vi "raise move v0.5.vi"(8 "error in (no error)":errorcluster) -> (0 "error out":errorcluster)   [LabVIEW 2019]
uses:
  <vilib>/Platform/TimedLoop/XDataNode/timing_clust.ctl
  <vilib>/Platform/TimedLoop/XDataNode/nitl_modes.ctl
  <vilib>/Platform/TimedLoop/XDataNode/wakeup.ctl
  FPGA_subVIs/low level/motor/motor enum.ctl
  <vilib>/platform/TimedLoop/XDataNode/XDataNode.xnode
  <vilib>/Platform/TimedLoop/XDataNode/XDNodeRunTimeDep.lvlib
  FPGA_subVIs/low level/motor/motor.lvlib
panel:
  out "Numeric":dbl
  out "-x":dbl
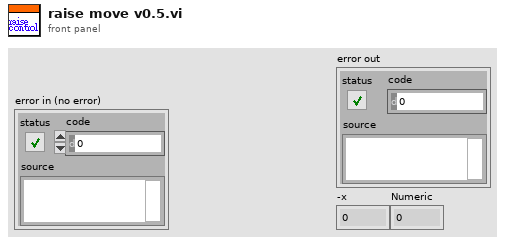
[diagram p1: front panel]
types:
  T1 = typedef "XDNodeRunTimeDep.lvlib/timing_clust.ctl" = cluster{"Expected End [f-1]":u64, "Actual End [f-1]":u64, "Finished Late? [f-1]":bool, "Expected End [i-1]":u64, "Actual End [i-1]":u64, "Finished Late? [i-1]":bool, "Expected Start [i]":u64, "Actual Start [i]":u64, "Expected Start [f]":u64, "Actual Start [f]":u64, "Source Name":string, "Structure Name":string, "Period":i64, "Deadline":i64, "Offset":i64, "Start":i64, "Priority":i32, "Timeout":i32, "Mode":T2, "Wakeup Reason":T3, "Error":errorcluster, "Source Type":string, "Secondary Source Type":string, "Global End Time":u64, "Global Start Time":u64, "Frame Duration":u64, "Iteration Duration":u64, "Assigned CPU":i32, "I/O Scan Engine Mode":u32}
  T2 = typedef "XDNodeRunTimeDep.lvlib/nitl_modes.ctl" = enum32{"No Change", "Process missed periods, maintain original phase", "Discard missed periods, maintain original phase", "Process missed periods, ignore original phase", "Discard missed periods, ignore original phase"}
  T3 = typedef "XDNodeRunTimeDep.lvlib/wakeup.ctl" = enum32{"Normal", "Aborted", "Asynchronous wakeup", "Timing source error", "Timed loop error", "Timeout"}
  T4 = typedef "my FPGA lib.lvlib/motor.lvlib/motor enum.ctl" = enum16{"M1", "M2", "M3", "M4"}
  T5 = cluster{"proportional gain (Kc)":dbl, "integral time (Ti, min)":dbl, "derivative time (Td, min)":dbl}
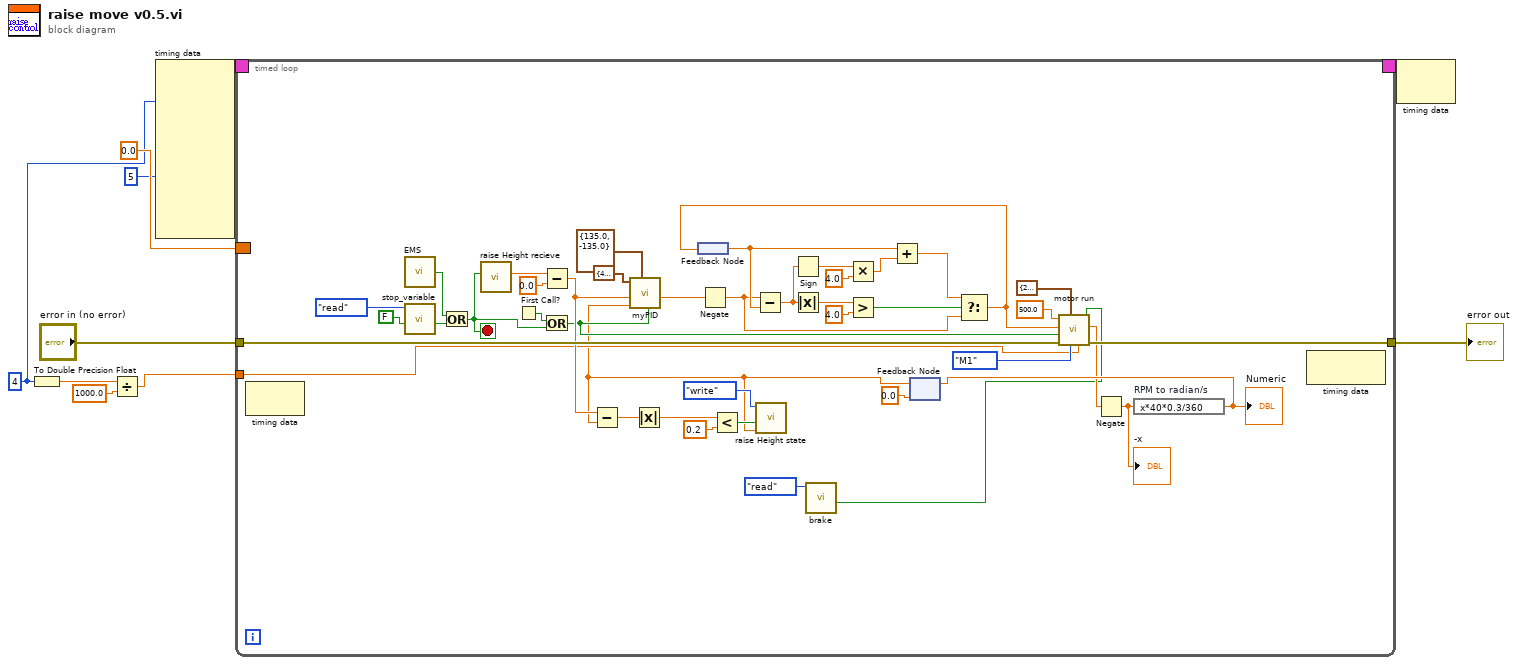
[diagram p0: block diagram]
diagram:
  w4 = i64 4 ("Period")
  n1 = To Double Precision Float(number=w4) -> (double precision float=w8:dbl)
  n2 = Divide(x=w8, y=1000.0) -> (x/y=w3:dbl)
  n3 = node-c288(w4, i64 5 ("Offset")) -> (w10:T1)  [unwired: 8 in]
  n4 = timed-loop {
    timing: w10 -> [_]
    timing-out: [_] -> w9
    tunnel: w3 -> [w18]
    tunnel: [w48] -> w6
    border: 0.0 -> [_]
    tunnel: "error in (no error)" -> [w34]
    stop <- w14 stop-if-true
    n5 = node-c288() -> ()  [unwired: 1 in, 1 out]
    n6 = call "EMS.vi"() -> ("A/DIO4 (Pin 19)"=w32:bool)
    n7 = call "stop_variable.vi"("Write"=FALSE, "Enum"=enum16{"read", "write"}."read") -> ("read"=w30:bool)  [unwired: 8 in, 1 out]
    n8 = Or(x=w32, y=w30) -> (x .or. y?=w14:bool)
    n9 = call "raise Height recieve.vi"("stop?"=w14) -> ("Height_cm"=w37:dbl)  [unwired: 9 in, 1 out]
    n10 = First Call?() -> (First Call?: T/F=w19:bool)
    n11 = Subtract(x=w37, y=0.0 ("x")) -> (x-y=w29:dbl)
    n12 = Or(x=w19, y=w14) -> (x .or. y?=w15:bool)
    n13 = feedback #1() -> (w44:dbl)
    n14 = call "brake.vi"("Enum"=enum16{"read", "write"}."read") -> ("read"=w12:bool)  [unwired: 9 in, 1 out]
    n15 = feedback #2(0.0) -> (w13:dbl)
    n16 = Subtract(x=w29, y=w13) -> (x-y=w28:dbl)
    n17 = call "myPID.vi"("s"=w15, "output range"=cluster{"output high":dbl, "output low":dbl} {"output high"=135.0, "output low"=-135.0}, "Processer"=w13, "setpoint"=w29, "PID"=cluster{"Kp":dbl, "Ki":dbl, "Kd":dbl} {"Kp"=45.0, "Ki"=0.0, "Kd"=0.0002}) -> ("out"=w49:dbl)  [unwired: 5 in, 1 out]
    n18 = Absolute Value(x=w28) -> (abs(x)=w27:dbl)
    n19 = Negate(x=w49) -> (-x=w39:dbl)
    n20 = Less?(x=w27, y=0.2) -> (x < y?=w24:bool)
    n21 = Subtract(x=w39, y=w44) -> (x-y=w38:dbl)
    n22 = call "raise Height state.vi"("Write Height"=w13, "Write"=w24, "Enum"=enum16{"read", "write"}."write") -> ()  [unwired: 7 in, 2 out]
    n23 = Sign(1:w38) -> (0:w43:dbl)
    n24 = Absolute Value(x=w38) -> (abs(x)=w47:dbl)
    n25 = Multiply(x=w43, y=4.0) -> (x*y=w41:dbl)
    n26 = Greater?(x=w47, y=4.0) -> (0:w45:bool)
    n27 = Add(x=w44, y=w41) -> (x+y=w40:dbl)
    n28 = Select(t=w40, s=w45, f=w39) -> (s? t:f=w21:dbl)
    n29 = feedback-in #1(w21) -> ()
    n30 = call "motor run.vi"("Motor.brake"=w12, "dt(s)"=w18, "motor select"=motor_enum."M1", "PID gains"=T5 {"proportional gain (Kc)"=20.0, "integral time (Ti, min)"=0.0, "derivative time (Td, min)"=0.0002}, "error in"=w34, "Reset"=w15, "speed RPM"=w21, "PWM frequence"=500.0) -> ("error out"=w48:errorcluster, "encoder"=w16:dbl)  [unwired: 2 out]
    n31 = Negate(x=w16) -> (-x=w50:dbl)
    "-x" <- w50
    n32 = expression code="x*40*0.3/360" "RPM to radian/s"(w50) -> (w35:dbl)
    "Numeric" <- w35
    n33 = feedback-in #2(w35) -> ()
    n34 = node-c288() -> ()  [unwired: 1 in, 1 out]
  }
  "error out" <- w6
  n35 = node-c288(w9) -> ()  [unwired: 1 out]
